vi "Post Step Read Holding Register.vi"(10 "Read Register Step Data":T1, 11 "Sequence Context In":refnum<k7>) -> (0 "error out":errorcluster, 1 "Read Data":dbl[](array[numeric]), 2 "Read Raw Data":u16[][](array[numeric]), 3 "Report Text":string)   [LabVIEW 2023, in "LTT_TeststandSteptypes.lvlib"]
uses:
  LTT_TeststandSteptypes.lvlib
  HardwareAbstractionLayer_LVOOP/Modbus/Modbus_class/Teststand Steptypes/Control/ReadRegisterSteptypeControl.ctl
  Control/TC FGV Action.ctl
  HardwareAbstractionLayer_LVOOP/Database/Database.lvclass
  HardwareAbstractionLayer_LVOOP/Database/SQL Public VI/Control/DB Options.ctl
  HardwareAbstractionLayer_LVOOP/Modbus/Modbus_class/Modbus.lvclass
panel:
  in  "error in":errorcluster
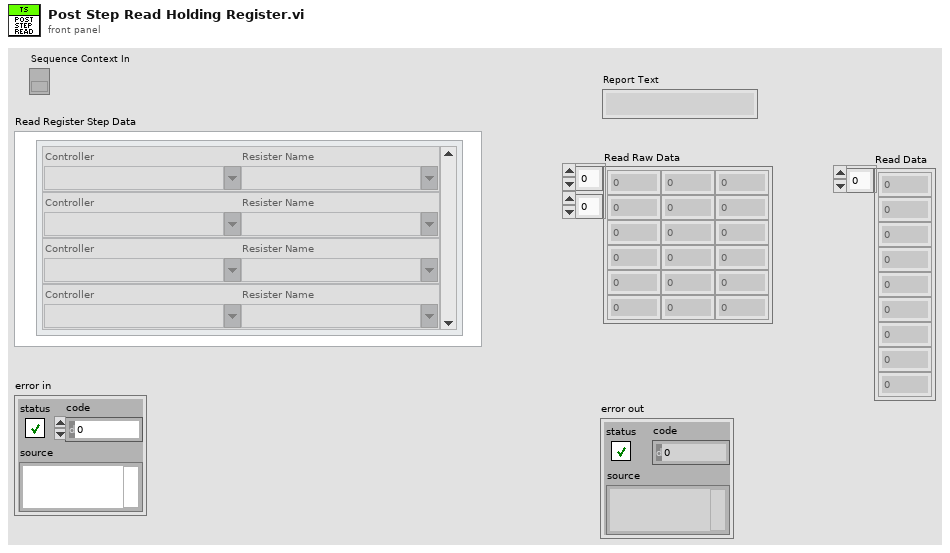
[diagram p1: front panel]
types:
  T1 = typedef "HardwareAbstractionLayer_LVOOP.lvlib/Modbus.lvclass/ReadRegisterSteptypeControl.ctl" = cluster{"Edit Controller":cluster{"Controller":string, "Resister Name":string}[]}
  T2 = typedef "HardwareAbstractionLayer_LVOOP.lvlib/Database.lvclass/DB Options.ctl" = enum16{"Init", "Select Data", "Insert Data", "Update Data", "Delete Data", "Execute Query", "Create Schema", "Create Table", "List Tables", "List Columns", "Close"}
  T3 = cluster{"Controller":string, "Resister Name":string}[]
  T4 = typedef "LTT_TeststandSteptypes.lvlib/TC FGV Action.ctl" = enum16{"Set", "Get"}
  T5 = typedef "HardwareAbstractionLayer_LVOOP.lvlib/Report.lvclass/Temperature LOG.ctl" = cluster{"TEST_MODE":string, "CYCLE_NUMBER":string, "TEMPERATURE":cluster{"LV_PPS_TEMPERATURE":dbl, "HV_PPS1_TEMPERATURE":dbl, "HV_PPS2_TEMPERATURE":dbl, "HV_PPS3_TEMPERATURE":dbl, "HV_PPS4_TEMPERATURE":dbl, "HV_PPS5_TEMPERATURE":dbl, "HV_PPS6_TEMPERATURE":dbl, "CHAMBER_TEMPERATURE":dbl, "LOAD_U1_TEMPERATURE":dbl, "LOAD_V1_TEMPERATURE":dbl, "LOAD_W1_TEMPERATURE":dbl, "LOAD_U2_TEMPERATURE":dbl, "LOAD_V2_TEMPERATURE":dbl, "LOAD_W2_TEMPERATURE":dbl, "LOAD_U3_TEMPERATURE":dbl, "LOAD_V3_TEMPERATURE":dbl, "LOAD_W3_TEMPERATURE":dbl}, "Temperature Inrange":cluster{"LVPPS_Trip?":bool, "HVPPS1_Trip?":bool, "HVPPS2_Trip?":bool, "HVPPS3_Trip?":bool, "HVPPS4_Trip?":bool, "HVPPS5_Trip?":bool, "HVPPS6_Trip?":bool, "Chamber_Trip?":bool}}
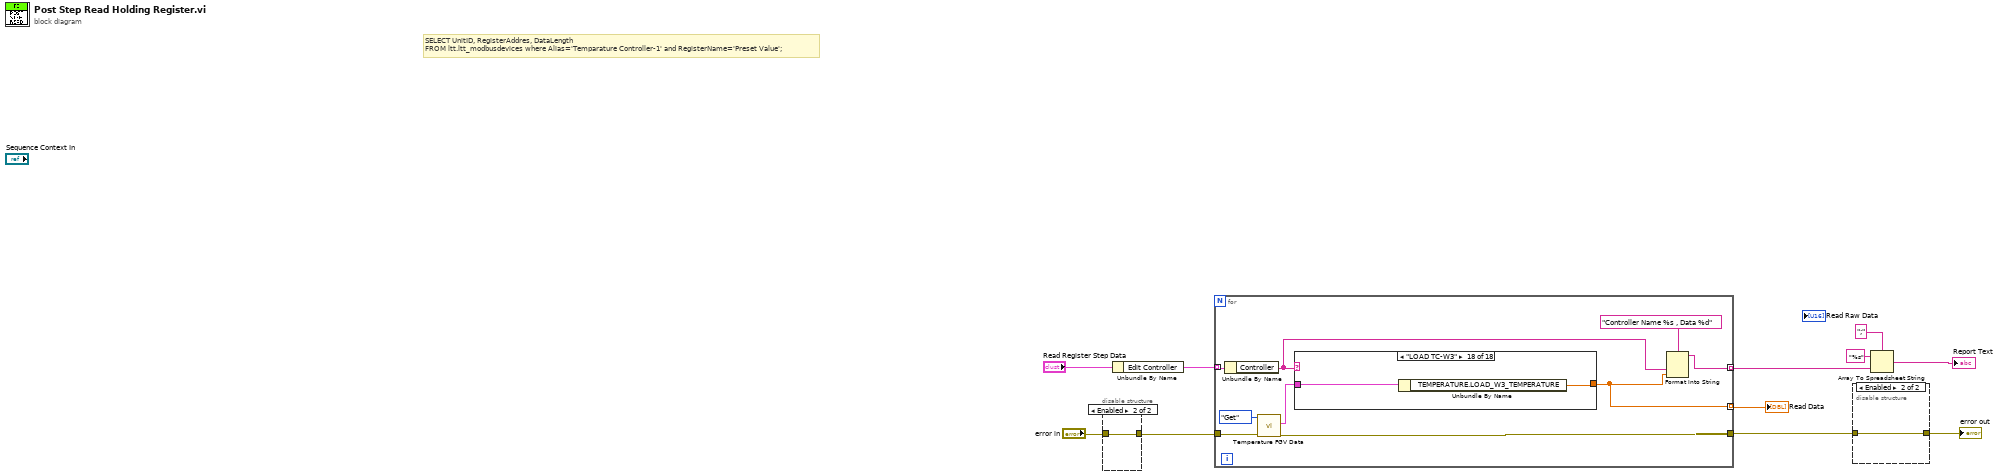
[diagram p0: block diagram]
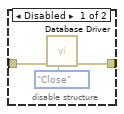
[diagram p2: hidden frame]
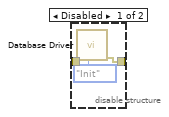
[diagram p3: hidden frame]
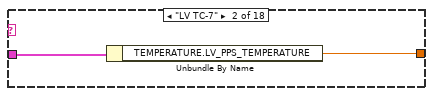
[diagram p5: hidden frame]
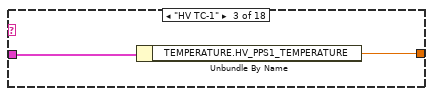
[diagram p6: hidden frame]
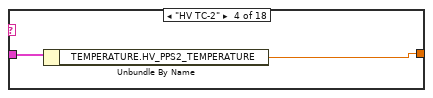
[diagram p7: hidden frame]
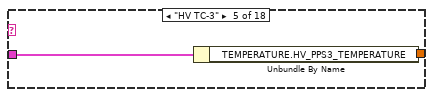
[diagram p8: hidden frame]
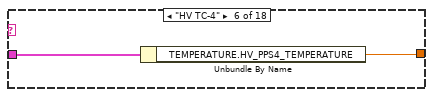
[diagram p9: hidden frame]
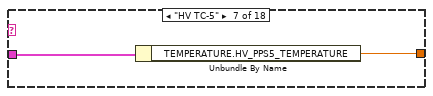
[diagram p10: hidden frame]
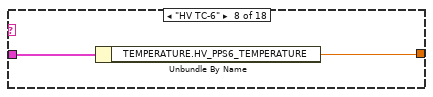
[diagram p11: hidden frame]
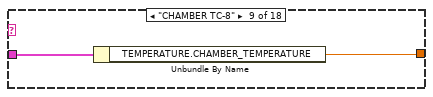
[diagram p12: hidden frame]
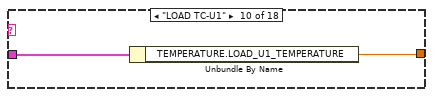
[diagram p13: hidden frame]
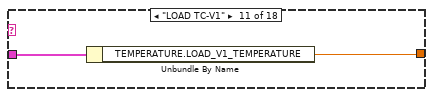
[diagram p14: hidden frame]
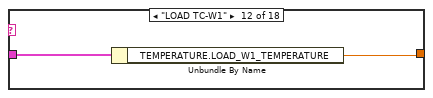
[diagram p15: hidden frame]
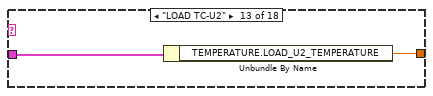
[diagram p16: hidden frame]
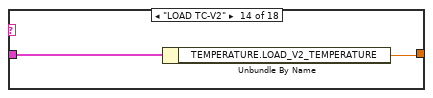
[diagram p17: hidden frame]
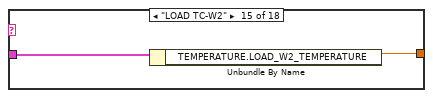
[diagram p18: hidden frame]
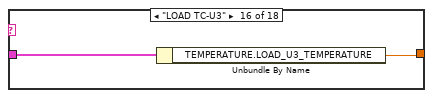
[diagram p19: hidden frame]
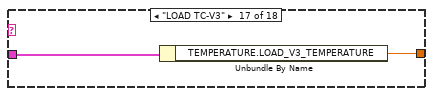
[diagram p20: hidden frame]
diagram:
  # "SELECT UnitID, RegisterAddres, DataLength\nFROM ltt.ltt_modbusdevices where Alias='Temparature Controller-1' and RegisterName='Preset Value';"
  n1 = disable-structure shown="Enabled" {
    disable-tunnel: "error in" -> [w13 w15]
    disable-tunnel: [w12 w15] -> w1
    frame Disabled {
      n2 = call "Database Driver.vi"("Options"=DB_Options."Init", "error in"=w13) -> ("error out"=w12:errorcluster)  [unwired: 6 in, 3 out]
    }
    frame Enabled {
    }
  }
  n3 = Unbundle By Name("Read Register Step Data") -> ("Edit Controller"=w2:T3)
  n4 = for {
    tunnel: w2 -> [w17] mode=indexing
    tunnel: [w23] -> w8 mode=indexing
    tunnel: w1 -> [w22]
    tunnel: [w20] -> w4
    tunnel: [w18] -> w3 mode=indexing
    n5 = Unbundle By Name(w17) -> ("Controller"=w16:string)
    n6 = call "Temperature FGV Data.vi"("error in"=w22, "Action"=TC_FGV_Action."Get") -> ("error out"=w20:errorcluster, "Temperature log Out"=w19:T5)  [unwired: 8 in]
    n7 = case shown="\"LOAD TC-W3\"" w16 {
      tunnel: w19 -> [_ w26 w28 w30 w32 w34 w36 w38 w40 w42 w44 w46 w48 w50 w52 w54 w56 w58]
      tunnel: [_ w25 w27 w29 w31 w33 w35 w37 w39 w41 w43 w45 w47 w49 w51 w53 w55 w57] -> w18
      frame Default {
      }
      frame "LV TC-7" {
        n8 = Unbundle By Name(w26) -> ("TEMPERATURE.LV_PPS_TEMPERATURE"=w25:dbl)
      }
      frame "HV TC-1" {
        n9 = Unbundle By Name(w28) -> ("TEMPERATURE.HV_PPS1_TEMPERATURE"=w27:dbl)
      }
      frame "HV TC-2" {
        n10 = Unbundle By Name(w30) -> ("TEMPERATURE.HV_PPS2_TEMPERATURE"=w29:dbl)
      }
      frame "HV TC-3" {
        n11 = Unbundle By Name(w32) -> ("TEMPERATURE.HV_PPS3_TEMPERATURE"=w31:dbl)
      }
      frame "HV TC-4" {
        n12 = Unbundle By Name(w34) -> ("TEMPERATURE.HV_PPS4_TEMPERATURE"=w33:dbl)
      }
      frame "HV TC-5" {
        n13 = Unbundle By Name(w36) -> ("TEMPERATURE.HV_PPS5_TEMPERATURE"=w35:dbl)
      }
      frame "HV TC-6" {
        n14 = Unbundle By Name(w38) -> ("TEMPERATURE.HV_PPS6_TEMPERATURE"=w37:dbl)
      }
      frame "CHAMBER TC-8" {
        n15 = Unbundle By Name(w40) -> ("TEMPERATURE.CHAMBER_TEMPERATURE"=w39:dbl)
      }
      frame "LOAD TC-U1" {
        n16 = Unbundle By Name(w42) -> ("TEMPERATURE.LOAD_U1_TEMPERATURE"=w41:dbl)
      }
      frame "LOAD TC-V1" {
        n17 = Unbundle By Name(w44) -> ("TEMPERATURE.LOAD_V1_TEMPERATURE"=w43:dbl)
      }
      frame "LOAD TC-W1" {
        n18 = Unbundle By Name(w46) -> ("TEMPERATURE.LOAD_W1_TEMPERATURE"=w45:dbl)
      }
      frame "LOAD TC-U2" {
        n19 = Unbundle By Name(w48) -> ("TEMPERATURE.LOAD_U2_TEMPERATURE"=w47:dbl)
      }
      frame "LOAD TC-V2" {
        n20 = Unbundle By Name(w50) -> ("TEMPERATURE.LOAD_V2_TEMPERATURE"=w49:dbl)
      }
      frame "LOAD TC-W2" {
        n21 = Unbundle By Name(w52) -> ("TEMPERATURE.LOAD_W2_TEMPERATURE"=w51:dbl)
      }
      frame "LOAD TC-U3" {
        n22 = Unbundle By Name(w54) -> ("TEMPERATURE.LOAD_U3_TEMPERATURE"=w53:dbl)
      }
      frame "LOAD TC-V3" {
        n23 = Unbundle By Name(w56) -> ("TEMPERATURE.LOAD_V3_TEMPERATURE"=w55:dbl)
      }
      frame "LOAD TC-W3" {
        n24 = Unbundle By Name(w58) -> ("TEMPERATURE.LOAD_W3_TEMPERATURE"=w57:dbl)
      }
    }
    n25 = Format Into String(format string="Controller Name %s , Data %d", w16, w18) -> (resulting string=w23:string)  [unwired: 2 in, 1 out]
  }
  "Read Data" <- w3
  n26 = disable-structure shown="Enabled" {
    disable-tunnel: w4 -> [w61 w62]
    disable-tunnel: [w60 w62] -> w10
    frame Disabled {
      n27 = call "Database Driver.vi"("Options"=DB_Options."Close", "error in"=w61) -> ("error out"=w60:errorcluster)  [unwired: 6 in, 3 out]
    }
    frame Enabled {
    }
  }
  "error out" <- w10
  n28 = Array To Spreadsheet String(delimiter (Tab)=";", array=w8, 3:"%s" ("format string")) -> (spreadsheet string=→"Report Text":string)
